vi "Split Waveform for Final Pulse Test.vi"(0 "Waveform In":waveform(dbl)={"t0"=timestamp(3433165898.5470004 s since 1904-01-01), "dt"=1e-05, "Y"=array[4250 elements]}, 5 "Final Threshold":dbl=2.5 format="%.2p", 7 "Samples before end":dbl=1000.0, 11 "error in (no error)":errorcluster) -> (4 "output waveform":waveform(dbl), 8 "Off for last 20%?":bool, 15 "error out":errorcluster)   [LabVIEW 2010]
uses:
  <vilib>/measure/mamon.llb/Trigger Detection for 1 Channel.vi
  <vilib>/Waveform/WDTOps.llb/WDT Get Waveform Subset DBL.vi
  <vilib>/measure/NI_MAPro.lvlib
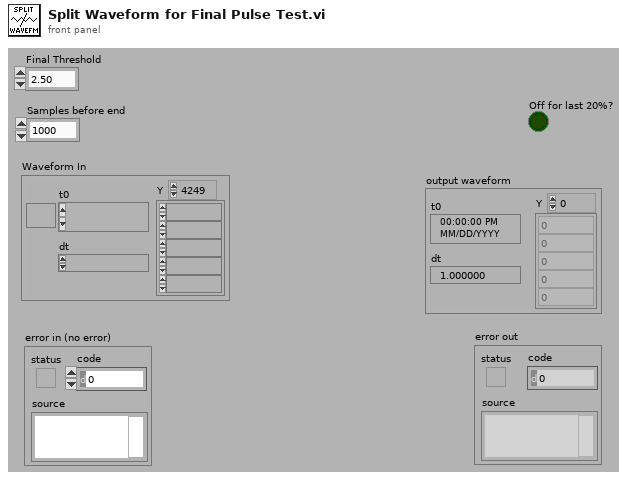
[diagram p1: front panel]
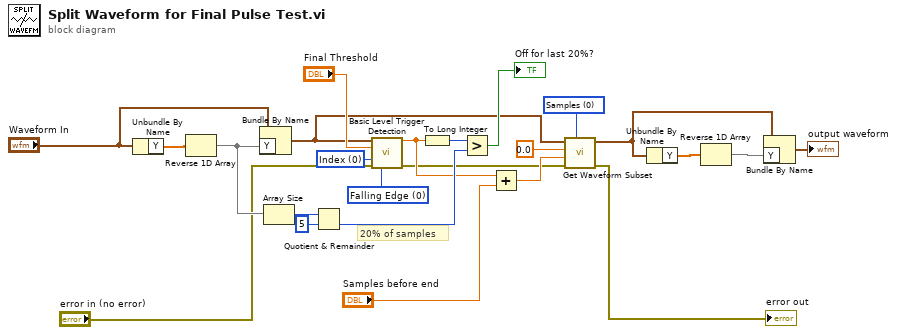
[diagram p0: block diagram]
diagram:
  w13 = u16 0 items=["Samples", "Relative Time"] ("start/duration format")
  w15 = u16 0 items=["Index", "Time"] ("location mode")
  w22 = u16 0 items=["Falling Edge", "Rising Edge"] ("trigger slope")
  # "20% of samples"
  n1 = Unbundle By Name("Waveform In") -> ("Y"=w1:dbl[])
  n2 = Reverse 1D Array(array=w1) -> (reversed array=w23:dbl[])
  n3 = Bundle By Name(cluster="Waveform In", "Y"=w23) -> (w14:waveform(dbl))
  n4 = Array Size(array=w23) -> (size(s)=w20:i32)
  n5 = Quotient & Remainder(x=w20, y=5) -> (floor(x/y)=w18:i32)  [unwired: 1 out]
  n6 = call-poly <vilib>:"Basic Level Trigger Detection.vi"("signal in"=w14, "level"="Final Threshold", "location mode"=w15, "error in (no error)"="error in (no error)", "trigger slope"=w22) -> ("trigger location"=w11:dbl, "error out"=w4:errorcluster)  [unwired: 8 in, 1 out]
  n7 = To Long Integer(number=w11) -> (32bit integer=w17:i32)
  n8 = Greater?(x=w17, y=w18) -> (0:→"Off for last 20%?":bool)
  n9 = Add(x=w11, y="Samples before end") -> (x+y=w10:dbl)
  n10 = call-poly <vilib>:"Get Waveform Subset.vi"("start/duration format"=w13, "error in (no error)"=w4, "duration"=w10, "start samples/time"=0.0, "waveform in"=w14) -> ("error out"=→"error out":errorcluster, "waveform out"=w6:waveform(dbl))  [unwired: 1 in, 2 out]
  n11 = Unbundle By Name(w6) -> ("Y"=w7:dbl[])
  n12 = Reverse 1D Array(array=w7) -> (reversed array=w8:dbl[])
  n13 = Bundle By Name(cluster=w6, "Y"=w8) -> (→"output waveform":waveform(dbl))
